vi "Global Obtain.vi"(8 "error in (no error)":errorcluster) -> (0 "error out":errorcluster, 1 "Created New?":bool, 3 "Global":refnum<k1>)   [LabVIEW 2022 SP3, in "Shared.lvlib"]
uses:
  Controls/Global.ctl
  Shared.lvlib
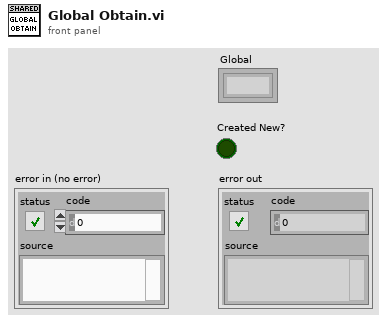
[diagram p1: front panel]
types:
  T1 = cluster{"ID":i32, "Name":string, "Parent":i32, "Queue":refnum<queue>, "Ini Path":path, "Ini Section":string, "VI Name":string, "VI Path":path, "VI Refnum":refnum<vi>, "Group":string}
  T2 = typedef "Shared.lvlib/Global.ctl" = cluster{"ID":i32, "Name":string, "Parent":i32, "Queue":refnum<queue>, "Ini Path":path, "Ini Section":string, "VI Name":string, "VI Path":path, "VI Refnum":refnum<vi>, "Group":string}
  T3 = cluster{"ID":i32, "Name":string, "Parent":i32, "Queue":refnum<queue>, "Ini Path":path, "Ini Section":string, "VI Name":string, "VI Path":path, "VI Refnum":refnum<vi>, "Group":string}[]
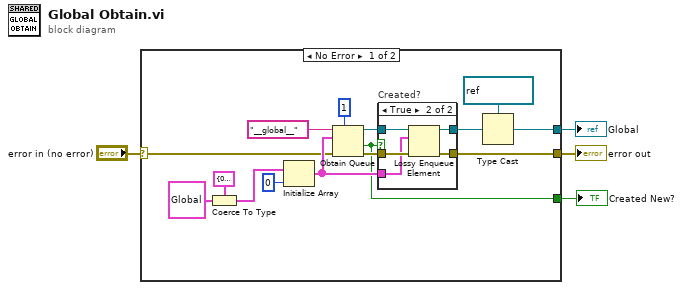
[diagram p0: block diagram]
diagram:
  n1 = case shown="No Error" "error in (no error)" {
    selector: "error in (no error)" -> [w11 w27]
    tunnel: [w10 w27] -> w3
    tunnel: [w7 _] -> w2
    tunnel: [w6 _] -> w1
    frame No Error {
      w8 = refnum<k1> refnum items=["Global"] ("Global")
      n2 = Coerce To Type(0:T2 {"ID"=0, "Name"="", "Parent"=0, "Queue"=refnum, "Ini Path"=path "", "Ini Section"="", "VI Name"="", "VI Path"=path "", "VI Refnum"=refnum, "Group"=""} ("Global"), 1:T1 {"ID"=0, "Name"="", "Parent"=0, "Queue"=refnum, "Ini Path"=path "", "Ini Section"="", "VI Name"="", "VI Path"=path "", "VI Refnum"=refnum, "Group"=""} ("Global")) -> (2:w12:T1)
      n3 = Initialize Array(w12, 0 ("dimension size")) -> (w14:T3)
      n4 = Obtain Queue(max queue size (-1, unlimited)=1, name (unnamed)="__global__", element data type=w14, error in (no error)=w11) -> (queue out=w17:refnum<queue>, created new?=w6:bool, error out=w16:errorcluster)  [unwired: 1 in]
      n5 = case "Created?" shown="True" w6 {
        tunnel: w17 -> [w21 w26]
        tunnel: w16 -> [w20 w25]
        tunnel: [w21 w24] -> w9
        tunnel: w14 -> [_ w23]
        tunnel: [w20 w22] -> w10
        frame False {
        }
        frame True {
          n6 = Lossy Enqueue Element(queue=w26, element=w23, error in (no error)=w25) -> (queue out=w24:refnum<queue>, error out=w22:errorcluster)  [unwired: 2 out]
        }
      }
      n7 = Type Cast(type=w8, x=w9) -> (*(type *) &x=w7:refnum<k1>)
    }
    frame Error {
    }
  }
  "error out" <- w3
  "Global" <- w2
  "Created New?" <- w1
